vi "SIM921_write.vi"(5 "File Reference":refnum<file>) -> ()   [LabVIEW 2019]
uses:
  Global/Global Variables/Data_Display_global.vi
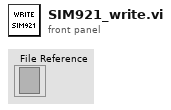
[diagram p1: front panel]
types:
  T1 = typedef "SIM921_resistance_Bridge_cluster.ctl" = cluster{"Resistance Ch1":dbl, "Update":bool}
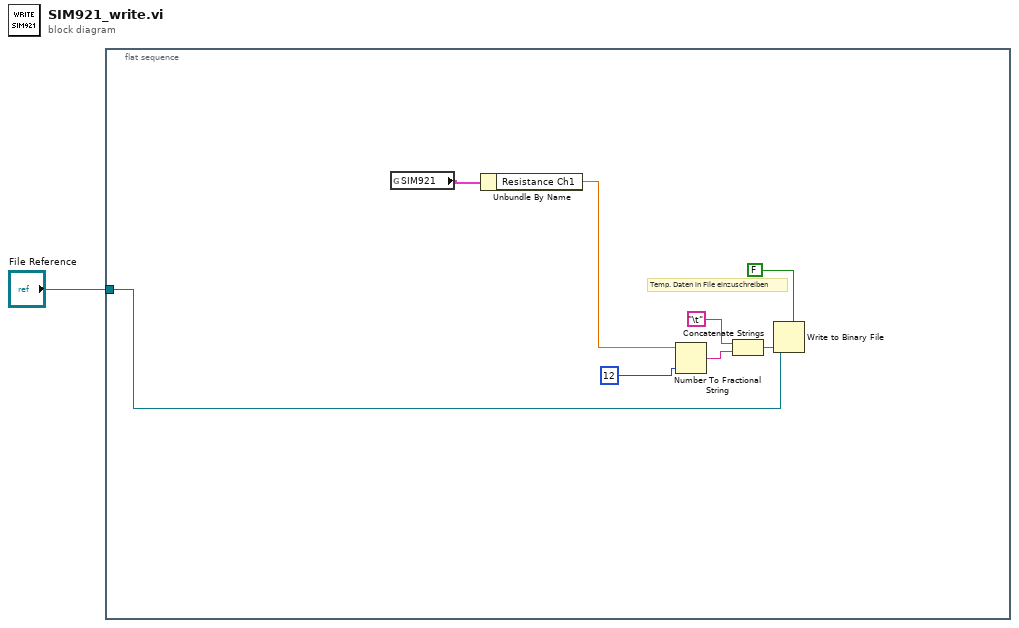
[diagram p0: block diagram]
diagram:
  n1 = flat-sequence {
    tunnel: "File Reference" -> [w2]
    frame #0 {
      # "Temp. Daten in File einzuschreiben"
      n2 = global read "Data_Display_global.vi" "SIM921"() -> (w4:T1)
      n3 = Unbundle By Name(w4) -> ("Resistance Ch1"=w3:dbl)
      n4 = Number To Fractional String(number=w3, precision (6)=i16 12) -> (F-format string=w5:string)  [unwired: 2 in]
      n5 = Concatenate Strings("\t", w5) -> (w9:string)
      n6 = Write to Binary File ("Write File")(file (use dialog)=w2, data=w9, 5:FALSE ("prepend array or string size? (T)")) -> ()  [unwired: 3 in, 3 out]
    }
  }
